vi "Лабораторная №1 Задание 3_5.vi"() -> ()   [LabVIEW 2017]
panel:
  in  "Умножение":dbl(knob) scale=0.0..10.0
  out "Индикатор":dbl(slide) scale=-1.0..1.0
  in  "Индикатор":dbl(knob) scale=-1.0..1.0
  in  "Frequency":dbl
  in  "stop":bool
  in  "Амплитуда":dbl(knob) scale=0.0..10.0
  out "Waveform Graph":dynamicdata(graph)
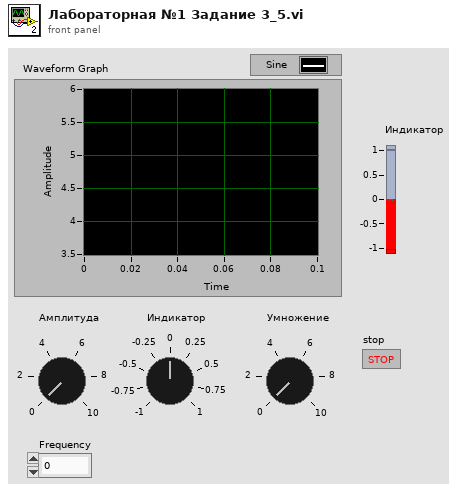
[diagram p1: front panel]
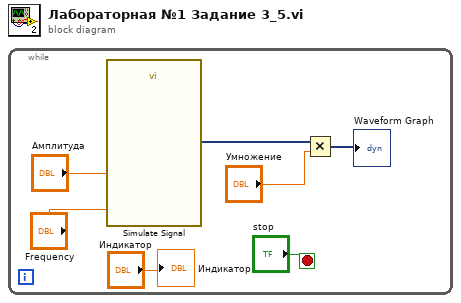
[diagram p0: block diagram]
diagram:
  n1 = while {
    stop <- "stop" stop-if-true
    n2 = call "Simulate Signal"("Frequency"="Frequency", "Amplitude"="Амплитуда") -> ("Sine"=w3:dynamicdata)  [unwired: 12 in, 1 out]
    n3 = Multiply(x=w3, y="Умножение") -> (x*y=→"Waveform Graph":dynamicdata)
    "Индикатор" <- "Индикатор"
  }
